vi "Fit Regularized IRF.vi"(6 "Weighted Fit? (T)":bool=TRUE, 8 "Error In":errorcluster, 9 "Time Constant":dbl, 10 "Intensity Array":dbl[](array[numeric]), 11 "t Array":dbl[](array[numeric])) -> (0 "Error Out":errorcluster, 1 "Fit Statistics":T1={"# Iterations"=0, "# Function Calls"=0, "Chi2"=0.0, "Chi2/DOF"=0.0, "Fit Convergence Criterion"=enum."Continue", "Gradient"=0.0, "|Delta Chi 2|"=0.0, "|Delta Chi 2|/Chi 2"=0.0, "Max |Delta a| /|a|"=0.0, "Lambda"=-1.0}, 2 "IRF Array":dbl[](array[numeric]), 3 "t Array":dbl[](array[numeric]))   [LabVIEW 2021, in "Fits.lvlib"]
doc: "Extract IRF from provided decay and time constant"
uses:
  Fits.lvlib
  Decay Convolution/LM model function and gradient (IRF deconvolution + 1-Exp).vi
  Decay Convolution/IRF Deconvolution Parameters.ctl
  Arrays/Arrays.lvlib
  My Fit Stopping Criteria.ctl
  Fit Statistics v3.ctl
  Convergence Criteria.ctl
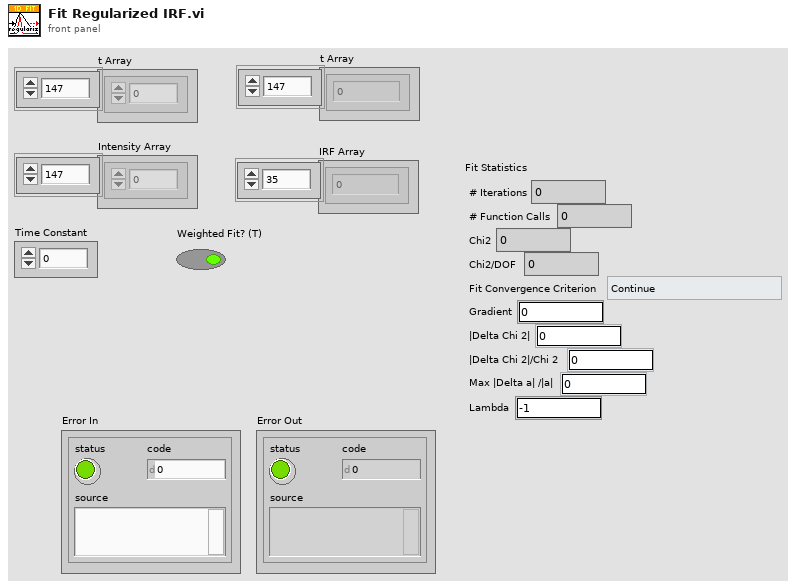
[diagram p1: front panel]
types:
  T1 = typedef "Fits.lvlib/Fit Statistics v2.ctl" = cluster{"# Iterations":i32, "# Function Calls":i32, "Chi2":dbl, "Chi2/DOF":dbl, "Fit Convergence Criterion":T2, "Gradient":dbl, "|Delta Chi 2|":dbl, "|Delta Chi 2|/Chi 2":dbl, "Max |Delta a| /|a|":dbl, "Lambda":dbl}
  T2 = typedef "Fits.lvlib/Convergence Criteria.ctl" = enum16{"Continue", "Tolerances Exceeded", "Max Time Exceeded", "Max Iterations Exceeded", "Max Function Evaluations Exceeded", "Scale Range Exceeded"}
  T3 = typedef "Fits.lvlib/My Fit Stopping Criteria.ctl" = cluster{"Max Iterations":i32, "Max Function Calls":i32, "Max Time":dbl[unit], "Function Tolerance":dbl, "Parameter Tolerance":dbl, "Gradient Tolerance":dbl, "Min Lambda":dbl, "Max Lambda":dbl, "Initial Tick Count":u32}
  T4 = cluster{"parameter minimum":dbl[], "parameter maximum":dbl[]}
  T5 = typedef "Fits.lvlib/IRF Deconvolution Parameters.ctl" = cluster{"IRF support":dbl[], "Lifetime":dbl}
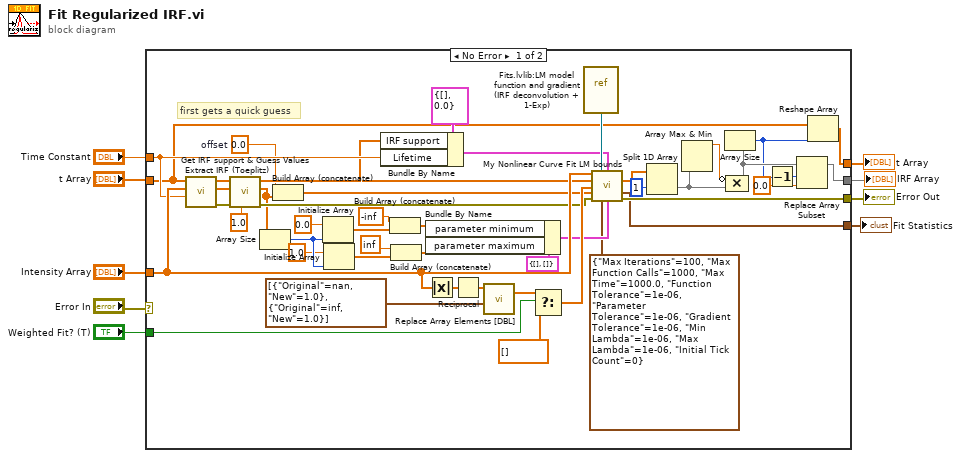
[diagram p0: block diagram]
diagram:
  n1 = case shown="No Error" "Error In" {
    selector: "Error In" -> [_ w56]
    tunnel: "Intensity Array" -> [w46 _]
    tunnel: "Time Constant" -> [w45 _]
    tunnel: "t Array" -> [w19 _]
    tunnel: [w33 w56] -> w6
    tunnel: "Weighted Fit? (T)" -> [w34 _]
    tunnel: [w16 _] -> w3
    tunnel: [w18 _] -> w2
    tunnel: [w22 _] -> w1
    frame No Error {
      w29 = 0.0  # offset
      # "first gets a quick guess"
      n2 = call "Extract IRF (Toeplitz).vi"("Time Constant"=w45, "Intensity Array"=w46, "t Array"=w19) -> ("Error Out"=w44:errorcluster, "IRF Array"=w11:dbl[], "t Array (dup)"=w43:dbl[])  [unwired: 5 in, 1 out]
      n3 = call "Get IRF support & Guess Values.vi"("Fraction of Original Support (0.7)"=1.0, "error in (no error)"=w44, "IRF Array in"=w11, "t Array in"=w43) -> ("error out"=w42:errorcluster, "IRF Array out"=w28:dbl[], "t Array out"=w31:dbl[])  [unwired: 5 in]
      n4 = Array Size(array=w28) -> (size(s)=w39:i32)
      n5 = Build Array (concatenate)(w29, w28) -> (w30:dbl[])
      n6 = Initialize Array(0.0 ("element"), w39) -> (w40:dbl[])
      n7 = Initialize Array(1.0 ("element"), w39) -> (w38:dbl[])
      n8 = Bundle By Name(cluster=T5 {"IRF support"=[], "Lifetime"=0.0} ("IRF"), "IRF support"=w31, "Lifetime"=w45) -> (w53:T5)
      n9 = Build Array (concatenate)(-inf ("element"), w40) -> (w27:dbl[])
      n10 = Build Array (concatenate)(inf ("element"), w38) -> (w25:dbl[])
      n11 = Bundle By Name(cluster=T4 {"parameter minimum"=[], "parameter maximum"=[]} ("parameter bounds"), "parameter minimum"=w27, "parameter maximum"=w25) -> (w36:T4)
      n12 = Absolute Value(x=w46) -> (abs(x)=w52:dbl[])
      n13 = Reciprocal(x=w52) -> (1/x=w51:dbl[])
      n14 = call "Replace Array Elements [DBL].vi"("Array of Replacement Pairs"=cluster{"Original":dbl, "New":dbl}[] [{"Original"=nan, "New"=1.0}, {"Original"=inf, "New"=1.0}], "Array"=w51) -> ("Array with Replacements"=w49:dbl[])  [unwired: 8 in, 1 out]
      n15 = Select(t=w49, s=w34, f=dbl[] [] ("Array with Replacements")) -> (s? t:f=w47:dbl[])
      n16 = vi-ref "Fits.lvlib:LM model function and gradient (IRF deconvolution + 1-Exp).vi"() -> (w55:refnum<vi>)
      n17 = call "My Nonlinear Curve Fit LM bounds.vi"("Y"=w46, "f(x,a)"=w55, "data"=w53, "X"=w19, "Weight"=w47, "initial parameters"=w30, "error in (no error)"=w42, "Termination Criteria"=T3 {"Max Iterations"=100, "Max Function Calls"=1000, "Max Time"=1000.0, "Function Tolerance"=1e-06, "Parameter Tolerance"=1e-06, "Gradient Tolerance"=1e-06, "Min Lambda"=1e-06, "Max Lambda"=1e-06, "Initial Tick Count"=0}, "parameter bounds"=w36) -> ("best fit parameters"=w32:dbl[], "Fit Statistics"=w22:T1, "error out"=w33:errorcluster)  [unwired: 1 in, 3 out]
      n18 = Split 1D Array(array=w32, index=1) -> (second subarray=w21:dbl[])  [unwired: 1 out]
      n19 = Array Max & Min(array=w21) -> (max value=w20:dbl)  [unwired: 3 out]
      n20 = Compound Arithmetic op=MULTIPLY(invert w20, w21) -> (w17:dbl[])
      n21 = Array Size(array=w17) -> (size(s)=w15:i32)
      n22 = Decrement(x=w15) -> (x-1=w14:i32)
      n23 = Replace Array Subset(array=w17, new element=0.0 ("new element/subarray"), index=w14) -> (w16:dbl[])
      n24 = Reshape Array(w19, w15) -> (w18:dbl[])
    }
    frame Error {
    }
  }
  "IRF Array" <- w3
  "Error Out" <- w6
  "t Array" <- w2
  "Fit Statistics" <- w1
